vi "搜索一维数组.vi"() -> ()   [LabVIEW 2018]
panel:
  out "字符串":string="注意：搜索时只会显示第一次搜索到元素的索引值，之后的索引值并不会显示。"
  in  "停止":bool
  out "元素索引":i32
  in  "开始索引(0)":i32
  in  "目标值":dbl
  in  "数组":dbl[](array[numeric])
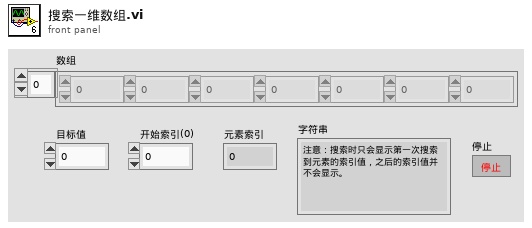
[diagram p1: front panel]
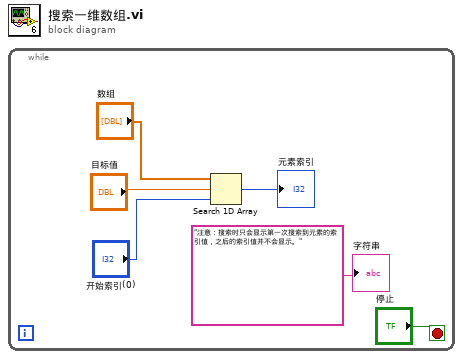
[diagram p0: block diagram]
diagram:
  n1 = while {
    stop <- "停止" stop-if-true
    n2 = Search 1D Array(1D array="数组", element="目标值", start index (0)="开始索引(0)") -> (index of element=→"元素索引":i32)
    "字符串" <- "注意：搜索时只会显示第一次搜索到元素的索引值，之后的索引值并不会显示。"
  }
